vi "Get Channel Data in By Channel ID.vi"(8 "error in (no error)":errorcluster, 9 "Channel IDs":T1[](array[typedef]) format="%.0x", 11 "Device Ref in":T1 format="%.0x") -> (0 "error out":errorcluster, 1 "Default Values":dbl[](array[numeric]), 2 "FIFO Indices":i32[](array[numeric]), 3 "Device Ref out":T1 format="%.0x", 4 "Channel Names":string[](array[string]))   [LabVIEW 2020, in "Routing and Faulting System Explorer.lvlib"]
uses:
  Routing and Faulting System Explorer.lvlib
  <vilib>/NI VeriStand/Custom Device API/Custom Device Item Ref.ctl
  <vilib>/NI VeriStand/Custom Device API/Custom Device API.lvlib
  <vilib>/NI VeriStand/Custom Device Tools/Custom Device Utility Library/Custom Device Utility Library.lvlib
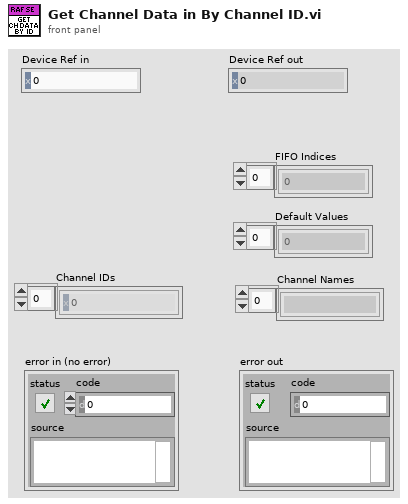
[diagram p1: front panel]
types:
  T1 = typedef "Custom Device API.lvlib/Custom Device Item Ref.ctl" = u64
  T2 = typedef "Custom Device API.lvlib/Custom Device Channel.ctl" = cluster{"Type":T3, "Units":string, "Default Value":dbl, "Faultable":bool, "Scalable":bool}
  T3 = typedef "Custom Device API.lvlib/Custom Device Channel Type.ctl" = enum16{"Input", "Output"}
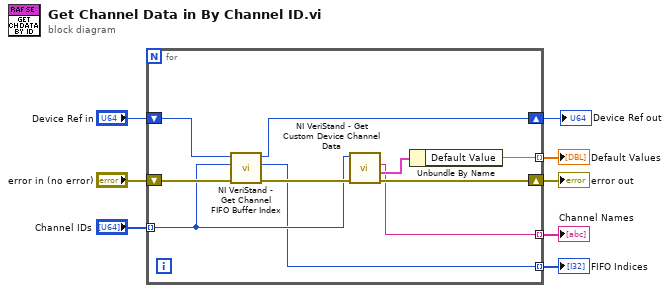
[diagram p0: block diagram]
diagram:
  n1 = for {
    shift-right: [w18] -> w7
    shift-left: "error in (no error)" -> [w14]
    tunnel: "Channel IDs" -> [w11] mode=indexing
    tunnel: [w16] -> w8 mode=indexing
    tunnel: [w15] -> w5 mode=indexing
    tunnel: [w10] -> w4 mode=indexing
    shift-right: [w9] -> w1
    shift-left: "Device Ref in" -> [w12]
    n2 = call <vilib>:"NI VeriStand - Get Channel FIFO Buffer Index.vi"("error in"=w14, "Channel Ref"=w11, "Device Ref in"=w12) -> ("error out"=w13:errorcluster, "Channel FIFO Buffer Index"=w10:i32, "Device Ref out"=w9:T1)  [unwired: 4 in, 2 out]
    n3 = call <vilib>:"NI VeriStand - Get Custom Device Channel Data.vi"("error in (no error)"=w13, "Channel Ref in"=w11) -> ("error out"=w18:errorcluster, "Channel"=w17:T2, "Channel Name"=w15:string)  [unwired: 4 in, 3 out]
    n4 = Unbundle By Name(w17) -> ("Default Value"=w16:dbl)
  }
  "Default Values" <- w8
  "error out" <- w7
  "FIFO Indices" <- w4
  "Channel Names" <- w5
  "Device Ref out" <- w1
